vi "CuLab_Gen_Waterfall.vi"(7 "WaterFall Config":cluster{"History":i32, "X Resolution":i32}={"History"=100, "X Resolution"=400000}, 8 "error in (no error)":errorcluster, 11 "Y":refnum<class "T1D_SGL.lvclass">) -> (0 "error IO":errorcluster, 1 "WaterFall":refnum<class "T2D_I16.lvclass">, 3 "WF Decimated":refnum<class "T1D_SGL.lvclass">)   [LabVIEW 2020]
uses:
  <vilib>/Ngene/CuLab - GPU Accelerated Toolkit/Toolkit/Low_Level/Tensor_Classes/T_Children/T1D/T1D_Children/T1D_SGL/T1D_SGL.lvclass
  C:/Program Files/National Instruments/LabVIEW 2020/vi.lib/Ngene/CuLab - GPU Accelerated Toolkit/Toolkit/Low_Level/Tensor_Classes/T_Children/T1D/T1D.lvclass
  <vilib>/Ngene/CuLab - GPU Accelerated Toolkit/Toolkit/Low_Level/Tensor_Classes/T_Children/T2D/T2D_Children/T2D_I16/T2D_I16.lvclass
  <vilib>/Ngene/CuLab - GPU Accelerated Toolkit/Toolkit/Low_Level/Tensor_Classes/T_Children/T2D/Controls/T2D_Dims.ctl
  <vilib>/Ngene/CuLab - GPU Accelerated Toolkit/Toolkit/Low_Level/Tensor_Classes/T_Children/T2D/Controls/T2D_Indices.ctl
  <vilib>/Ngene/CuLab - GPU Accelerated Toolkit/Toolkit/API/Signal Processing/Signal Operation/Decimate (single shot) adaptive/CU_Decimate_Single_Shot_Adaptive_T1D_SGL.vi
  <vilib>/Ngene/CuLab - GPU Accelerated Toolkit/Toolkit/Low_Level/Tensor_Classes/T_Children/T2D/T2D_Children/T2D_I16/Create.vi
  <vilib>/Ngene/CuLab - GPU Accelerated Toolkit/Toolkit/API/Numeric/Conversion  (API)/I16/CU_To_I16_T1D.vi
  <vilib>/Ngene/CuLab - GPU Accelerated Toolkit/Toolkit/CuLab.lvlib
  C:/Program Files/National Instruments/LabVIEW 2020/vi.lib/Ngene/CuLab - GPU Accelerated Toolkit/Toolkit/Low_Level/Tensor_Classes/Tensor.lvclass
  C:/Program Files/National Instruments/LabVIEW 2020/vi.lib/Ngene/CuLab - GPU Accelerated Toolkit/Toolkit/Low_Level/Tensor_Classes/T_Children/T1D/T1D_Children/T1D_SGL/T1D_SGL.lvclass
  <vilib>/Ngene/CuLab - GPU Accelerated Toolkit/Toolkit/API/Array/Replace Array Subset (API)/CU_Replace_Array_Subset_2D_1D/CU_Replace_Array_Subset_2D_1D_I16.vi
  <vilib>/Ngene/CuLab - GPU Accelerated Toolkit/Toolkit/API/Array/Replace Array Subset (API)/CU_Replace_Array_Subset_2D_2D/CU_Replace_Array_Subset_2D_2D_I16.vi
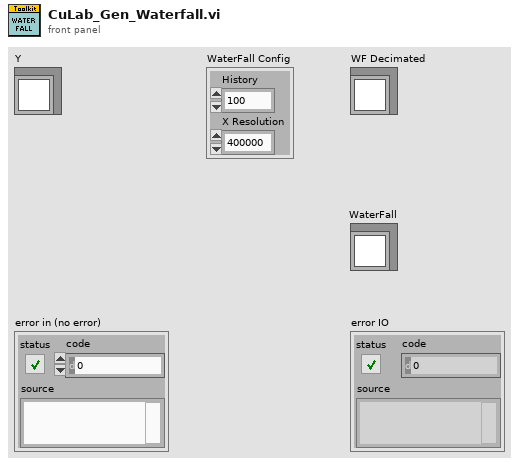
[diagram p1: front panel]
types:
  T1 = typedef "CuLab.lvlib/T2D_Dims.ctl" = cluster{"H":i32, "W":i32}
  T2 = typedef "CuLab.lvlib/T2D_Indices.ctl" = cluster{"i":i32, "j":i32}
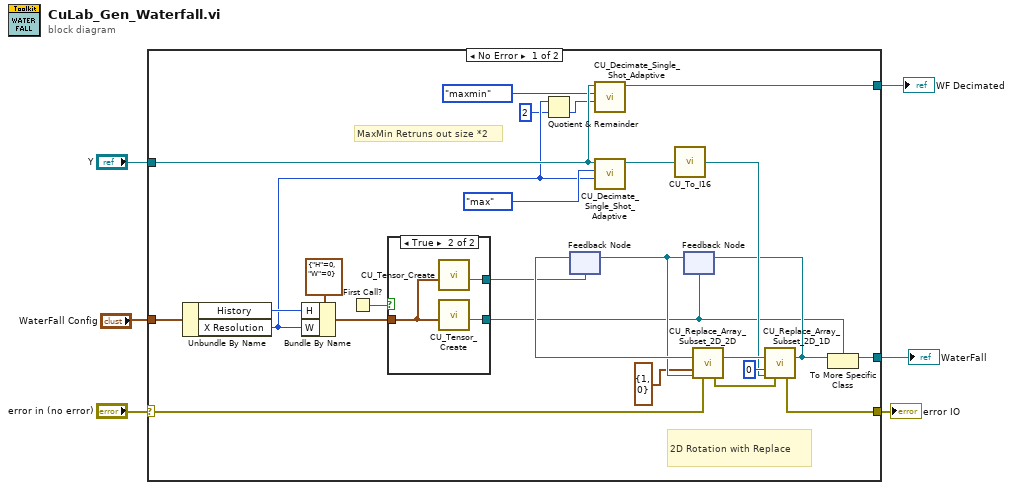
[diagram p0: block diagram]
diagram:
  n1 = case shown="No Error" "error in (no error)" {
    selector: "error in (no error)" -> [w16 w36]
    tunnel: "WaterFall Config" -> [w32 _]
    tunnel: "Y" -> [w12 _]
    tunnel: [w18 _] -> w4
    tunnel: [w9 _] -> w2
    tunnel: [w14 w36] -> w1
    frame No Error {
      # "MaxMin Retruns out size *2"
      # "2D Rotation with Replace"
      n2 = Unbundle By Name(w32) -> ("History"=w25:i32, "X Resolution"=w11:i32)
      n3 = Bundle By Name(cluster=T1 {"H"=0, "W"=0} ("T2D_Dims"), "H"=w25, "W"=w11) -> (w26:T1)
      n4 = First Call?() -> (First Call?: T/F=w24:bool)
      n5 = case shown="True" w24 {
        tunnel: [_ w35] -> w17
        tunnel: w26 -> [_ w34]
        tunnel: [_ w33] -> w22
        frame False {
        }
        frame True {
          n6 = call-poly <vilib>:"CU_Tensor_Create.vi"("T2D_Dims"=w34) -> ("T2D_I16 out"=w33:refnum<class "T2D_I16.lvclass">)  [unwired: 9 in, 1 out]
          n7 = call-poly <vilib>:"CU_Tensor_Create.vi"("T2D_Dims"=w34) -> ("T2D_I16 out"=w35:refnum<class "T2D_I16.lvclass">)  [unwired: 9 in, 1 out]
        }
      }
      n8 = Quotient & Remainder(x=w11, y=2) -> (floor(x/y)=w7:i32)  [unwired: 1 out]
      n9 = feedback #1(w22) -> (w31:refnum<class "T2D_I16.lvclass">)
      n10 = call-poly <vilib>:"CU_Decimate_Single_Shot_Adaptive.vi"("output size"=w7, "operation"=enum16{"avg", "min", "max", "maxmin"}."maxmin" ("operation 2"), "X"=w12) -> ("Decimated Array"=w9:refnum<class "T1D_SGL.lvclass">)  [unwired: 7 in, 1 out]
      n11 = call-poly <vilib>:"CU_Decimate_Single_Shot_Adaptive.vi"("output size"=w11, "operation"=enum16{"avg", "min", "max", "maxmin"}."max" ("operation 2"), "X"=w12) -> ("Decimated Array"=w13:refnum<class "T1D_SGL.lvclass">)  [unwired: 7 in, 1 out]
      n12 = call-poly <vilib>:"CU_To_I16.vi"("Tensor in"=w13) -> ("Dest out"=w21:refnum<class "T1D_I16.lvclass">)  [unwired: 13 in, 1 out]
      n13 = feedback #2(w17) -> (w30:refnum<class "T2D_I16.lvclass">)
      n14 = feedback-in #1(w30) -> ()
      n15 = call-poly <vilib>:"CU_Replace_Array_Subset_2D_2D.vi"("Tensor in"=w31, "Indices"=T2 {"i"=1, "j"=0}, "Sub Tensor"=w30, "error in (no error)"=w16) -> ("Tensor Out"=w29:refnum<class "T2D_I16.lvclass">, "error out"=w15:errorcluster)  [unwired: 10 in]
      n16 = call-poly <vilib>:"CU_Replace_Array_Subset_2D_1D.vi"("Tensor in"=w29, "index"=0, "Sub Tensor"=w21, "error in (no error)"=w15) -> ("Tensor Out"=w19:refnum<class "T2D_I16.lvclass">, "error out"=w14:errorcluster)  [unwired: 10 in]
      n17 = feedback-in #2(w19) -> ()
      n18 = To More Specific Class(target class=w17, reference=w19) -> (specific class reference=w18:refnum<class "T2D_I16.lvclass">)  [unwired: 1 in, 1 out]
    }
    frame Error {
    }
  }
  "WaterFall" <- w4
  "WF Decimated" <- w2
  "error IO" <- w1
